vi "CaseRegister2.vi"() -> ()   [LabVIEW 2021]
panel:
  out "String 3":string
  in  "String 2":string
  out "String":string
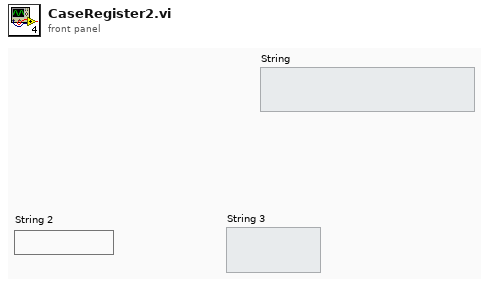
[diagram p1: front panel]
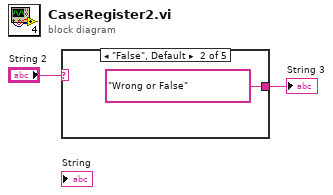
[diagram p0: block diagram]
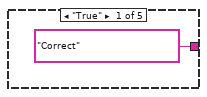
[diagram p2: hidden frame]
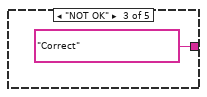
[diagram p3: hidden frame]
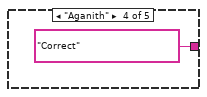
[diagram p4: hidden frame]
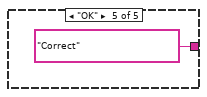
[diagram p5: hidden frame]
diagram:
  n1 = case shown="\"False\", Default" "String 2" {
    tunnel: ["Correct" "Wrong or False" "Correct" "Correct" "Correct"] -> w1
    frame "True" {
    }
    frame "False", Default {
    }
    frame "NOT OK" {
    }
    frame "Aganith" {
    }
    frame "OK" {
    }
  }
  "String 3" <- w1
